vi "DigitalOutput.vi"() -> ()   [LabVIEW 2014]
panel:
  in  "stop":bool
  in  "Freio":bool
  in  "Motor":bool
  out "Freio":bool
  out "Motor":bool
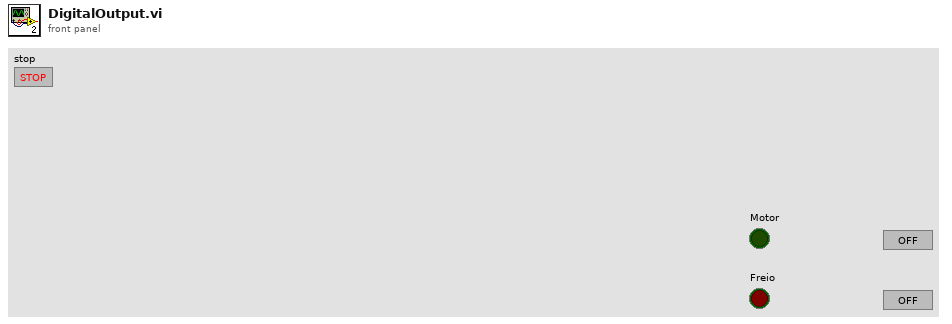
[diagram p1: front panel]
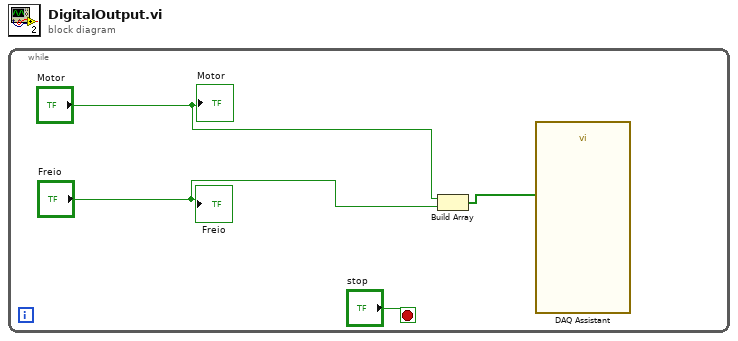
[diagram p0: block diagram]
diagram:
  n1 = while {
    stop <- "stop" stop-if-true
    n2 = Build Array("Motor", "Freio") -> (w1:bool[])
    n3 = call "DAQ Assistant"("data"=w1) -> ()  [unwired: 17 in, 2 out]
    "Motor" <- "Motor"
    "Freio" <- "Freio"
  }
